vi "ForceSettingsWrite.vi"(10 "Function":string(combo)="0" caption="Combo Box") -> (1 "k":dbl format="%#_13g", 2 "Setpoint":dbl format="%#_13g")   [LabVIEW 2023]
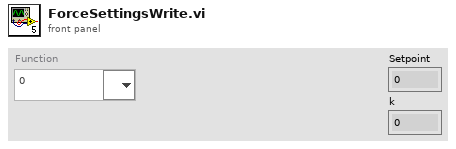
[diagram p1: front panel]
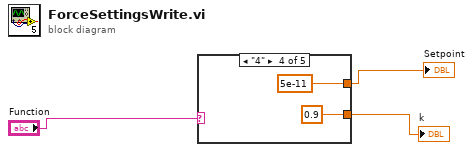
[diagram p0: block diagram]
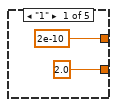
[diagram p2: hidden frame]
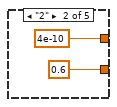
[diagram p3: hidden frame]
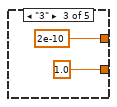
[diagram p4: hidden frame]
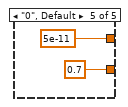
[diagram p5: hidden frame]
diagram:
  n1 = case shown="\"4\"" "Function" {
    tunnel: [2.0 0.6 1.0 0.9 0.7] -> w2
    tunnel: [2e-10 4e-10 2e-10 5e-11 5e-11] -> w1
    frame "1" {
    }
    frame "2" {
    }
    frame "3" {
    }
    frame "4" {
    }
    frame "0", Default {
    }
  }
  "Setpoint" <- w1
  "k" <- w2
